vi "parallel_loop.vi"() -> ()   [LabVIEW 2021]
panel:
  out "Array":dbl[](array[numeric])
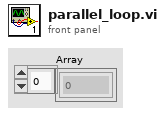
[diagram p1: front panel]
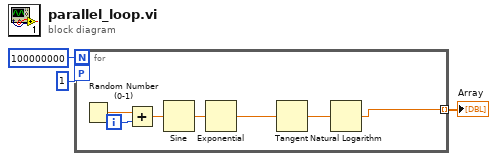
[diagram p0: block diagram]
diagram:
  n1 = for {
    N: 100000000 -> [_]
    workers-P: 1 -> [_]
    tunnel: [w4] -> w1 mode=indexing
    i -> [w7]
    n2 = Random Number (0-1)() -> (number: 0 to 1=w5:dbl)
    n3 = Add(x=w5, y=w7) -> (x+y=w6:dbl)
    n4 = Sine(x=w6) -> (sin(x)=w9:dbl)
    n5 = Exponential(1:w9) -> (0:w10:dbl)
    n6 = Tangent(1:w10) -> (0:w8:dbl)
    n7 = Natural Logarithm(1:w8) -> (0:w4:dbl)
  }
  "Array" <- w1
